vi "Simulate Signal Noise.vi"(8 "error in (no error)":errorcluster) -> (0 "error out":errorcluster, 1 "voltage noise":dbl, 3 "current noise":dbl)   [LabVIEW 2023, in "Simulated-PowerModule.lvlib" / "Simulated-PowerModule.lvclass"]
uses:
  Simulated-PowerModule.lvclass
  <vilib>/measure/NI_MABase.lvlib
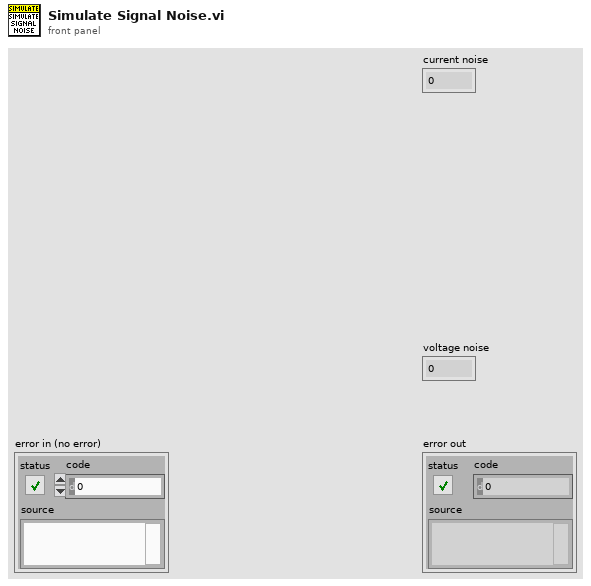
[diagram p1: front panel]
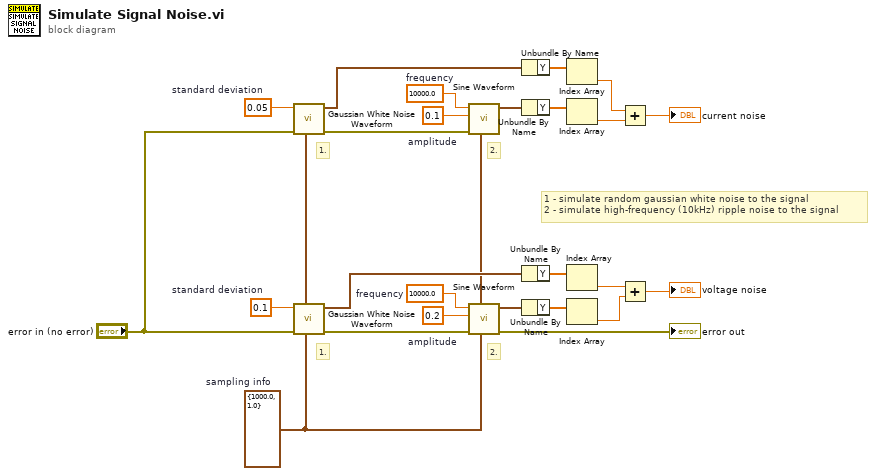
[diagram p0: block diagram]
diagram:
  w19 = 0.05  # standard deviation
  w16 = 10000.0  # frequency
  w17 = 0.1  # amplitude
  w13 = 10000.0  # frequency
  w12 = 0.2  # amplitude
  w9 = 0.1  # standard deviation
  w21 = cluster{"Fs":dbl, "#s":dbl} {"Fs"=1000.0, "#s"=1.0}  # sampling info
  # "2."
  # "1."
  # "1 - simulate random gaussian white noise to the signal\n2 - simulate high-frequency (10kHz) ripple noise to the signal"
  # "2."
  # "1."
  n1 = call <vilib>:"Gaussian White Noise Waveform.vi"("sampling info"=w21, "error in (no error)"="error in (no error)", "standard deviation"=w19) -> ("error out"=w20:errorcluster, "signal out"=w8:waveform(dbl))  [unwired: 7 in]
  n2 = call <vilib>:"Gaussian White Noise Waveform.vi"("sampling info"=w21, "error in (no error)"="error in (no error)", "standard deviation"=w9) -> ("error out"=w10:errorcluster, "signal out"=w24:waveform(dbl))  [unwired: 7 in]
  n3 = call <vilib>:"Sine Waveform.vi"("sampling info"=w21, "error in (no error)"=w20, "amplitude"=w17, "frequency"=w16) -> ("signal out"=w23:waveform(dbl))  [unwired: 6 in, 1 out]
  n4 = call <vilib>:"Sine Waveform.vi"("sampling info"=w21, "error in (no error)"=w10, "amplitude"=w12, "frequency"=w13) -> ("error out"=→"error out":errorcluster, "signal out"=w14:waveform(dbl))  [unwired: 6 in]
  n5 = Unbundle By Name(w8) -> ("Y"=w4:dbl[])
  n6 = Unbundle By Name(w23) -> ("Y"=w22:dbl[])
  n7 = Unbundle By Name(w24) -> ("Y"=w25:dbl[])
  n8 = Unbundle By Name(w14) -> ("Y"=w15:dbl[])
  n9 = Index Array(array=w4) -> (element=w3:dbl)  [unwired: 1 in]
  n10 = Index Array(array=w22) -> (element=w6:dbl)  [unwired: 1 in]
  n11 = Index Array(array=w25) -> (element=w2:dbl)  [unwired: 1 in]
  n12 = Index Array(array=w15) -> (element=w7:dbl)  [unwired: 1 in]
  n13 = Add(x=w3, y=w6) -> (x+y=→"current noise":dbl)
  n14 = Add(x=w2, y=w7) -> (x+y=→"voltage noise":dbl)
